vi "Unlock Data.vi"(8 "error in (no error)":errorcluster, 9 "Datum Type":variant, 10 "Datum Name":string, 11 "IModel in":refnum<class "IModel.lvclass">) -> (0 "error out":errorcluster, 3 "IModel out":refnum<class "IModel.lvclass">)   [LabVIEW 2019, in "IModel.lvlib" / "IModel.lvclass"]
uses:
  <vilib>/gpm_packages/@cs/mva-core/Source/IModel/IModel/IModel.lvclass
  C:/Program Files/National Instruments/LabVIEW 2019/vi.lib/gpm_packages/@cs/mva-core/Source/IObserver/IObserver/IObserver.lvclass
  <vilib>/gpm_packages/@cs/mva-core/Source/IObserver/IObserver/IObserver.lvclass/IObserver.ctl
  <vilib>/gpm_packages/@cs/mva-core/Source/IModel/IModel/IModel.lvclass/IModel.ctl
  <vilib>/gpm_packages/@cs/mva-core/Source/IMediator/IMediator Messages/Unlock Publication Msg/Unlock Publication Msg.lvclass/Unlock Publication Msg.ctl
  <vilib>/gpm_packages/@cs/actor-framework-messages/Source/RoundTripMessage/RoundTripMessage.lvclass/RoundTripMessage.ctl
  <vilib>/ActorFramework/Message Enqueuer/Message Enqueuer.lvclass/Message Enqueuer.ctl
  <vilib>/gpm_packages/@cs/actor-framework-messages/Source/RoundTripMessage/Return Round-Trip Message.vi
  <vilib>/ActorFramework/Message Enqueuer/Enqueue.vi
  <vilib>/gpm_packages/@cs/mva-core/Source/IMediator/IMediator Messages/Unlock Publication Msg/Unlock Publication Msg.lvclass
  C:/Program Files/National Instruments/LabVIEW 2019/vi.lib/gpm_packages/@cs/actor-framework-messages/Source/RoundTripMessage/RoundTripMessage.lvclass
  <vilib>/gpm_packages/@cs/actor-framework-messages/Source/RoundTripMessage/RoundTripMessage.lvclass
  C:/Program Files/National Instruments/LabVIEW 2019/vi.lib/ActorFramework/Message/Message.lvclass
  <vilib>/ActorFramework/Message Priority Queue/Priority Enqueue.vi
  <vilib>/gpm_packages/@cs/mva-core/Source/IObserver/IObserver/IObserver.lvclass
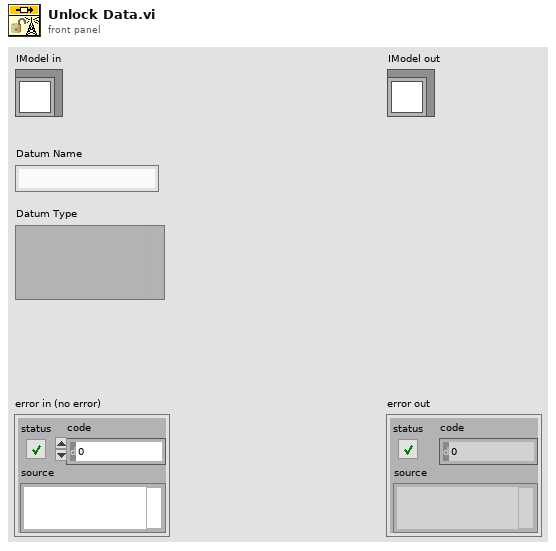
[diagram p1: front panel]
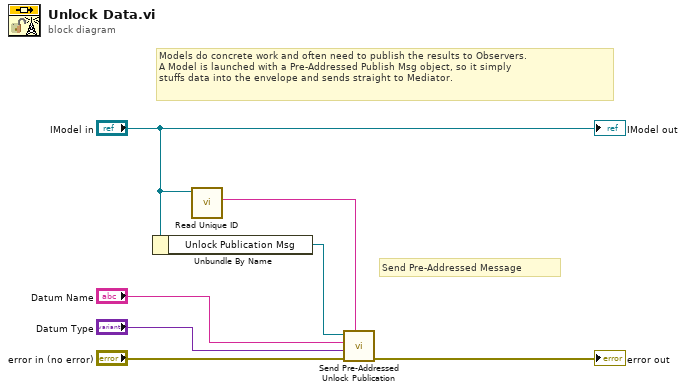
[diagram p0: block diagram]
diagram:
  # "Models do concrete work and often need to publish the results to Observers.\nA Model is launched with a Pre-Addressed Publish Msg object, so it simply\nstuffs data into the envelope and sends straight to Mediator."
  # "Send Pre-Addressed Message"
  n1 = Unbundle By Name("IModel in") -> ("Unlock Publication Msg"=w7:refnum<class "Unlock Publication Msg.lvclass">)
  n2 = call <vilib>:"Read Unique ID.vi"("IObserver In"="IModel in") -> ("Unique ID"=w1:string)  [unwired: 10 in]
  n3 = call <vilib>:"Send Pre-Addressed Unlock Publication.vi"("Publisher ID"=w1, "error in (no error)"="error in (no error)", "Data to Publish"="Datum Type", "Datum Name"="Datum Name", "Unlock Publication Msg"=w7) -> ("error out"=→"error out":errorcluster)  [unwired: 6 in]
  "IModel out" <- "IModel in"
